vi "Launcher.vi"() -> ()   [LabVIEW 2019]
uses:
  6 SEMESTRE/MICROPROCESADORES_AVANZADOS/P5_P2/INTERFACE_LABVIEW/INTERFACE UI Data.ctl
  Serial Devices/Serial Devices.lvclass
  C:/Program Files (x86)/National Instruments/LabVIEW 2019/vi.lib/ActorFramework/Actor/Actor.lvclass
  Serial Devices/Serial Devices.lvclass/Serial Devices.ctl
  Serial Devices/Write BRAND SELECTED.vi
  Serial Devices/Write SIMULATED_.vi
  Serial Devices/Write COM SELECTED.vi
  <vilib>/ActorFramework/Actor/Actor.lvclass
panel:
  in  "UI Data IN":T1
  in  "BRAND SELECTED":enum16{"NXP", "CYPRESS", "SIMULATED"}(ring)
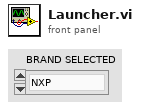
[diagram p1: front panel]
types:
  T1 = typedef "INTERFACE UI Data.ctl" = cluster{"Com":refnum<visa-resource-name>}
  T2 = enum8{"Enabled", "Disabled", "Disabled and Grayed Out"}
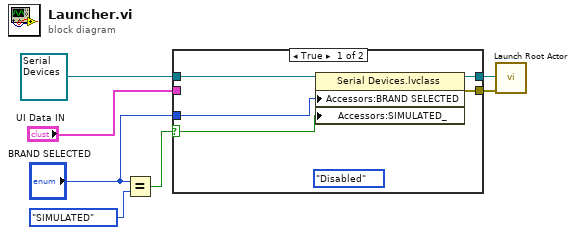
[diagram p0: block diagram]
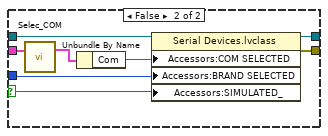
[diagram p2: hidden frame]
diagram:
  n1 = Equal?(x="BRAND SELECTED", y=enum16{"NXP", "CYPRESS", "SIMULATED"}."SIMULATED") -> (x = y?=w4:bool)
  n2 = case shown="True" w4 {
    selector: w4 -> [w9 w17]
    tunnel: refnum<class "Serial Devices.lvclass"> refnum ("Serial Devices.lvlib:Serial Devices.lvclass") -> [w12 w20]
    tunnel: [w11 w19] -> w7
    tunnel: [w10 w18] -> w6
    tunnel: "BRAND SELECTED" -> [w8 w13]
    tunnel: "UI Data IN" -> [_ w15]
    frame True {
      (unwired) T2."Disabled" ("Disabled")
      n3 = property class="Serial Devices.lvclass"(reference=w12, "Accessors:BRAND SELECTED"=w8, "Accessors:SIMULATED_"=w9) -> (reference out=w11:refnum<class "Serial Devices.lvclass">, error out=w10:errorcluster)  [unwired: 1 in]
    }
    frame False {
      n4 = call "Selec_COM.vi"("UI Data IN"=w15) -> ("UI Data OUT"=w16:T1)  [unwired: 10 in]
      n5 = Unbundle By Name(w16) -> ("Com"=w14:refnum<visa-resource-name>)
      n6 = property class="Serial Devices.lvclass"(reference=w20, "Accessors:COM SELECTED"=w14, "Accessors:BRAND SELECTED"=w13, "Accessors:SIMULATED_"=w17) -> (reference out=w19:refnum<class "Serial Devices.lvclass">, error out=w18:errorcluster)  [unwired: 1 in]
    }
  }
  n7 = call <vilib>:"Launch Root Actor.vi"("error in (no error)"=w6, "Actor"=w7) -> ()  [unwired: 8 in, 2 out]
